vi "Stop.vi"(8 "Error Input":errorcluster caption="Error In", 9 "TaskId":string, 10 "SessionId":string, 11 "LiteAgentSDK Input":refnum<k24>) -> (0 "Error Output":errorcluster caption="Error Out", 3 "LiteAgentSDK Output":refnum<k24>)   [LabVIEW 2017, in "LiteAgentSDK.lvlib"]
uses:
  LiteAgentSDK.lvlib
  C:/Users/Jan/Projects/LiteAgentSDK-LabVIEW/Source/Bin/LiteAgentSDK.LabVIEW.dll
  Bin/LiteAgentSDK.LabVIEW.dll
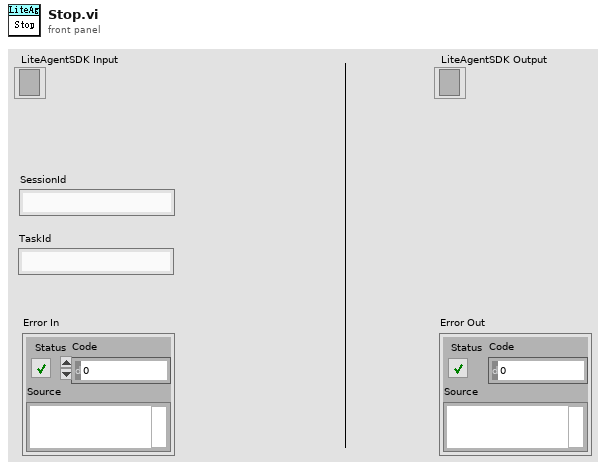
[diagram p1: front panel]
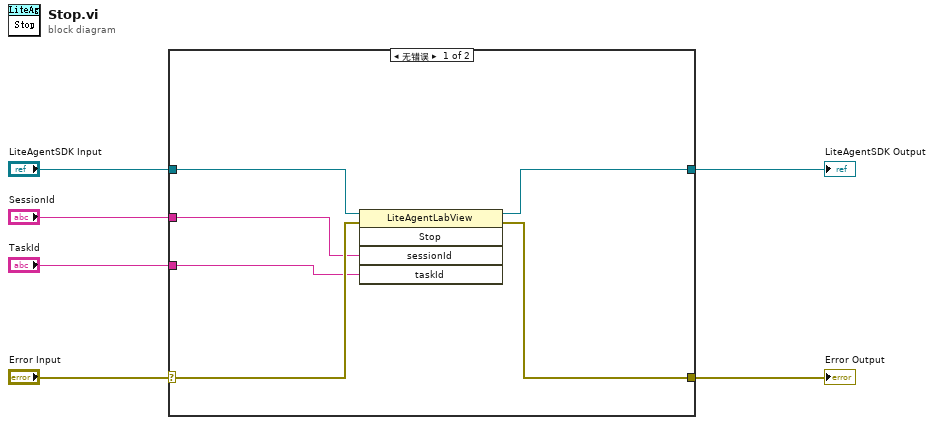
[diagram p0: block diagram]
diagram:
  n1 = case shown="无错误" "Error Input" {
    selector: "Error Input" -> [w12 w13]
    tunnel: "LiteAgentSDK Input" -> [w11 w14]
    tunnel: [w10 w14] -> w1
    tunnel: [w9 w13] -> w5
    tunnel: "SessionId" -> [w8 _]
    tunnel: "TaskId" -> [w7 _]
    frame No Error {
      n2 = invoke on="调用节点" class="LiteAgentLabView" method="Stop"(reference=w11, error in=w12, "sessionId"=w8, "taskId"=w7) -> (reference out=w10:refnum<k24>, error out=w9:errorcluster)  [unwired: 1 in, 3 out]
    }
    frame Error {
    }
  }
  "Error Output" <- w5
  "LiteAgentSDK Output" <- w1
